vi "ConvertUnitsToCounts.vi"(8 "error in (no error)":errorcluster, 10 "Coordinates.Units":T2, 11 "XYStage in":refnum<class "XYStage.lvclass">) -> (0 "error out":errorcluster, 2 "Coordinates.Counts":T1, 3 "XYStage out":refnum<class "XYStage.lvclass">)   [LabVIEW 2017, in "XYStage.lvclass"]
uses:
  XYStage.lvclass
  Typedefs/Coordinates.Units--Cluster.ctl
  Typedefs/Coordinates.Counts--Cluster.ctl
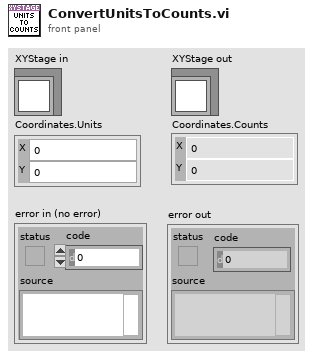
[diagram p1: front panel]
types:
  T1 = typedef "XYStage.lvclass/Coordinates.Counts--Cluster.ctl" = cluster{"X":i32, "Y":i32}
  T2 = typedef "XYStage.lvclass/Coordinates.Units--Cluster.ctl" = cluster{"X":dbl, "Y":dbl}
  T3 = typedef "XYStage.lvclass/Configuration--Cluster.ctl" = cluster{"Serial Number":string, "X Axis":string, "Y Axis":string, "Real-World Units":string, "Counts per Unit":u32}
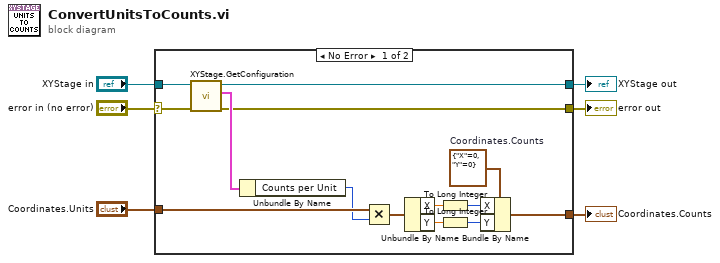
[diagram p0: block diagram]
diagram:
  n1 = case shown="No Error" "error in (no error)" {
    selector: "error in (no error)" -> [w19 w22]
    tunnel: [w8 w22] -> w5
    tunnel: [w9 w21] -> w3
    tunnel: "XYStage in" -> [w20 w21]
    tunnel: "Coordinates.Units" -> [w17 _]
    tunnel: [w7 _] -> w1
    frame No Error {
      w15 = T1 {"X"=0, "Y"=0}  # Coordinates.Counts
      n2 = call "XYStage.GetConfiguration.vi"("error in (no error)"=w19, "XYStage"=w20) -> ("error out"=w8:errorcluster, "Configuration"=w18:T3, "XYStage out"=w9:refnum<class "XYStage.lvclass">)  [unwired: 7 in]
      n3 = Unbundle By Name(w18) -> ("Counts per Unit"=w16:u32)
      n4 = Multiply(x=w17, y=w16) -> (x*y=w14:T2)
      n5 = Unbundle By Name(w14) -> ("X"=w13:dbl, "Y"=w11:dbl)
      n6 = To Long Integer(number=w13) -> (32bit integer=w12:i32)
      n7 = To Long Integer(number=w11) -> (32bit integer=w10:i32)
      n8 = Bundle By Name(cluster=w15, "X"=w12, "Y"=w10) -> (w7:T1)
    }
    frame Error {
    }
  }
  "error out" <- w5
  "XYStage out" <- w3
  "Coordinates.Counts" <- w1
